vi "Read Line Rate - Returns Default Value.vi"() -> ()   [LabVIEW 2017, in "Cobertura.Tests.lvlib" / "Class.lvlib"]
uses:
  Class.lvlib
  Cobertura/Class/Class.lvclass/Class.ctl
  Cobertura/Class/Read Line Rate.vi
  <vilib>/PNR/Transparent Assertions/Transparent Assertions/Transparent Assertions.lvlib
  Cobertura/Class/Class.lvclass
panel:
  out "error out":errorcluster
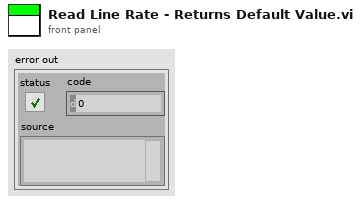
[diagram p1: front panel]
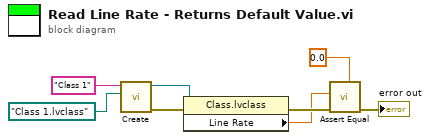
[diagram p0: block diagram]
diagram:
  n1 = call "Create.vi"("Filename"=path "Class 1.lvclass", "Name"="Class 1") -> ("error out"=w7:errorcluster, "Class"=w6:refnum<class "Class.lvclass">)  [unwired: 8 in]
  n2 = property class="Class.lvclass"(reference=w6, error in=w7) -> (error out=w5:errorcluster, "Line Rate"=w4:dbl)  [unwired: 1 out]
  n3 = call <vilib>:"Assert Equal.vi"("Expected"=0.0 ("Line Rate"), "error in (no error)"=w5, "Actual"=w4) -> ("error out"=→"error out":errorcluster)  [unwired: 8 in]
